vi "Config_Global.vi"() -> ()   [LabVIEW 2014]
panel:
  in  "Pod 3":T1
  in  "Pod 2":T1
  in  "Pod 1":T1
  in  "General":T2
  in  "Pod 0":T1
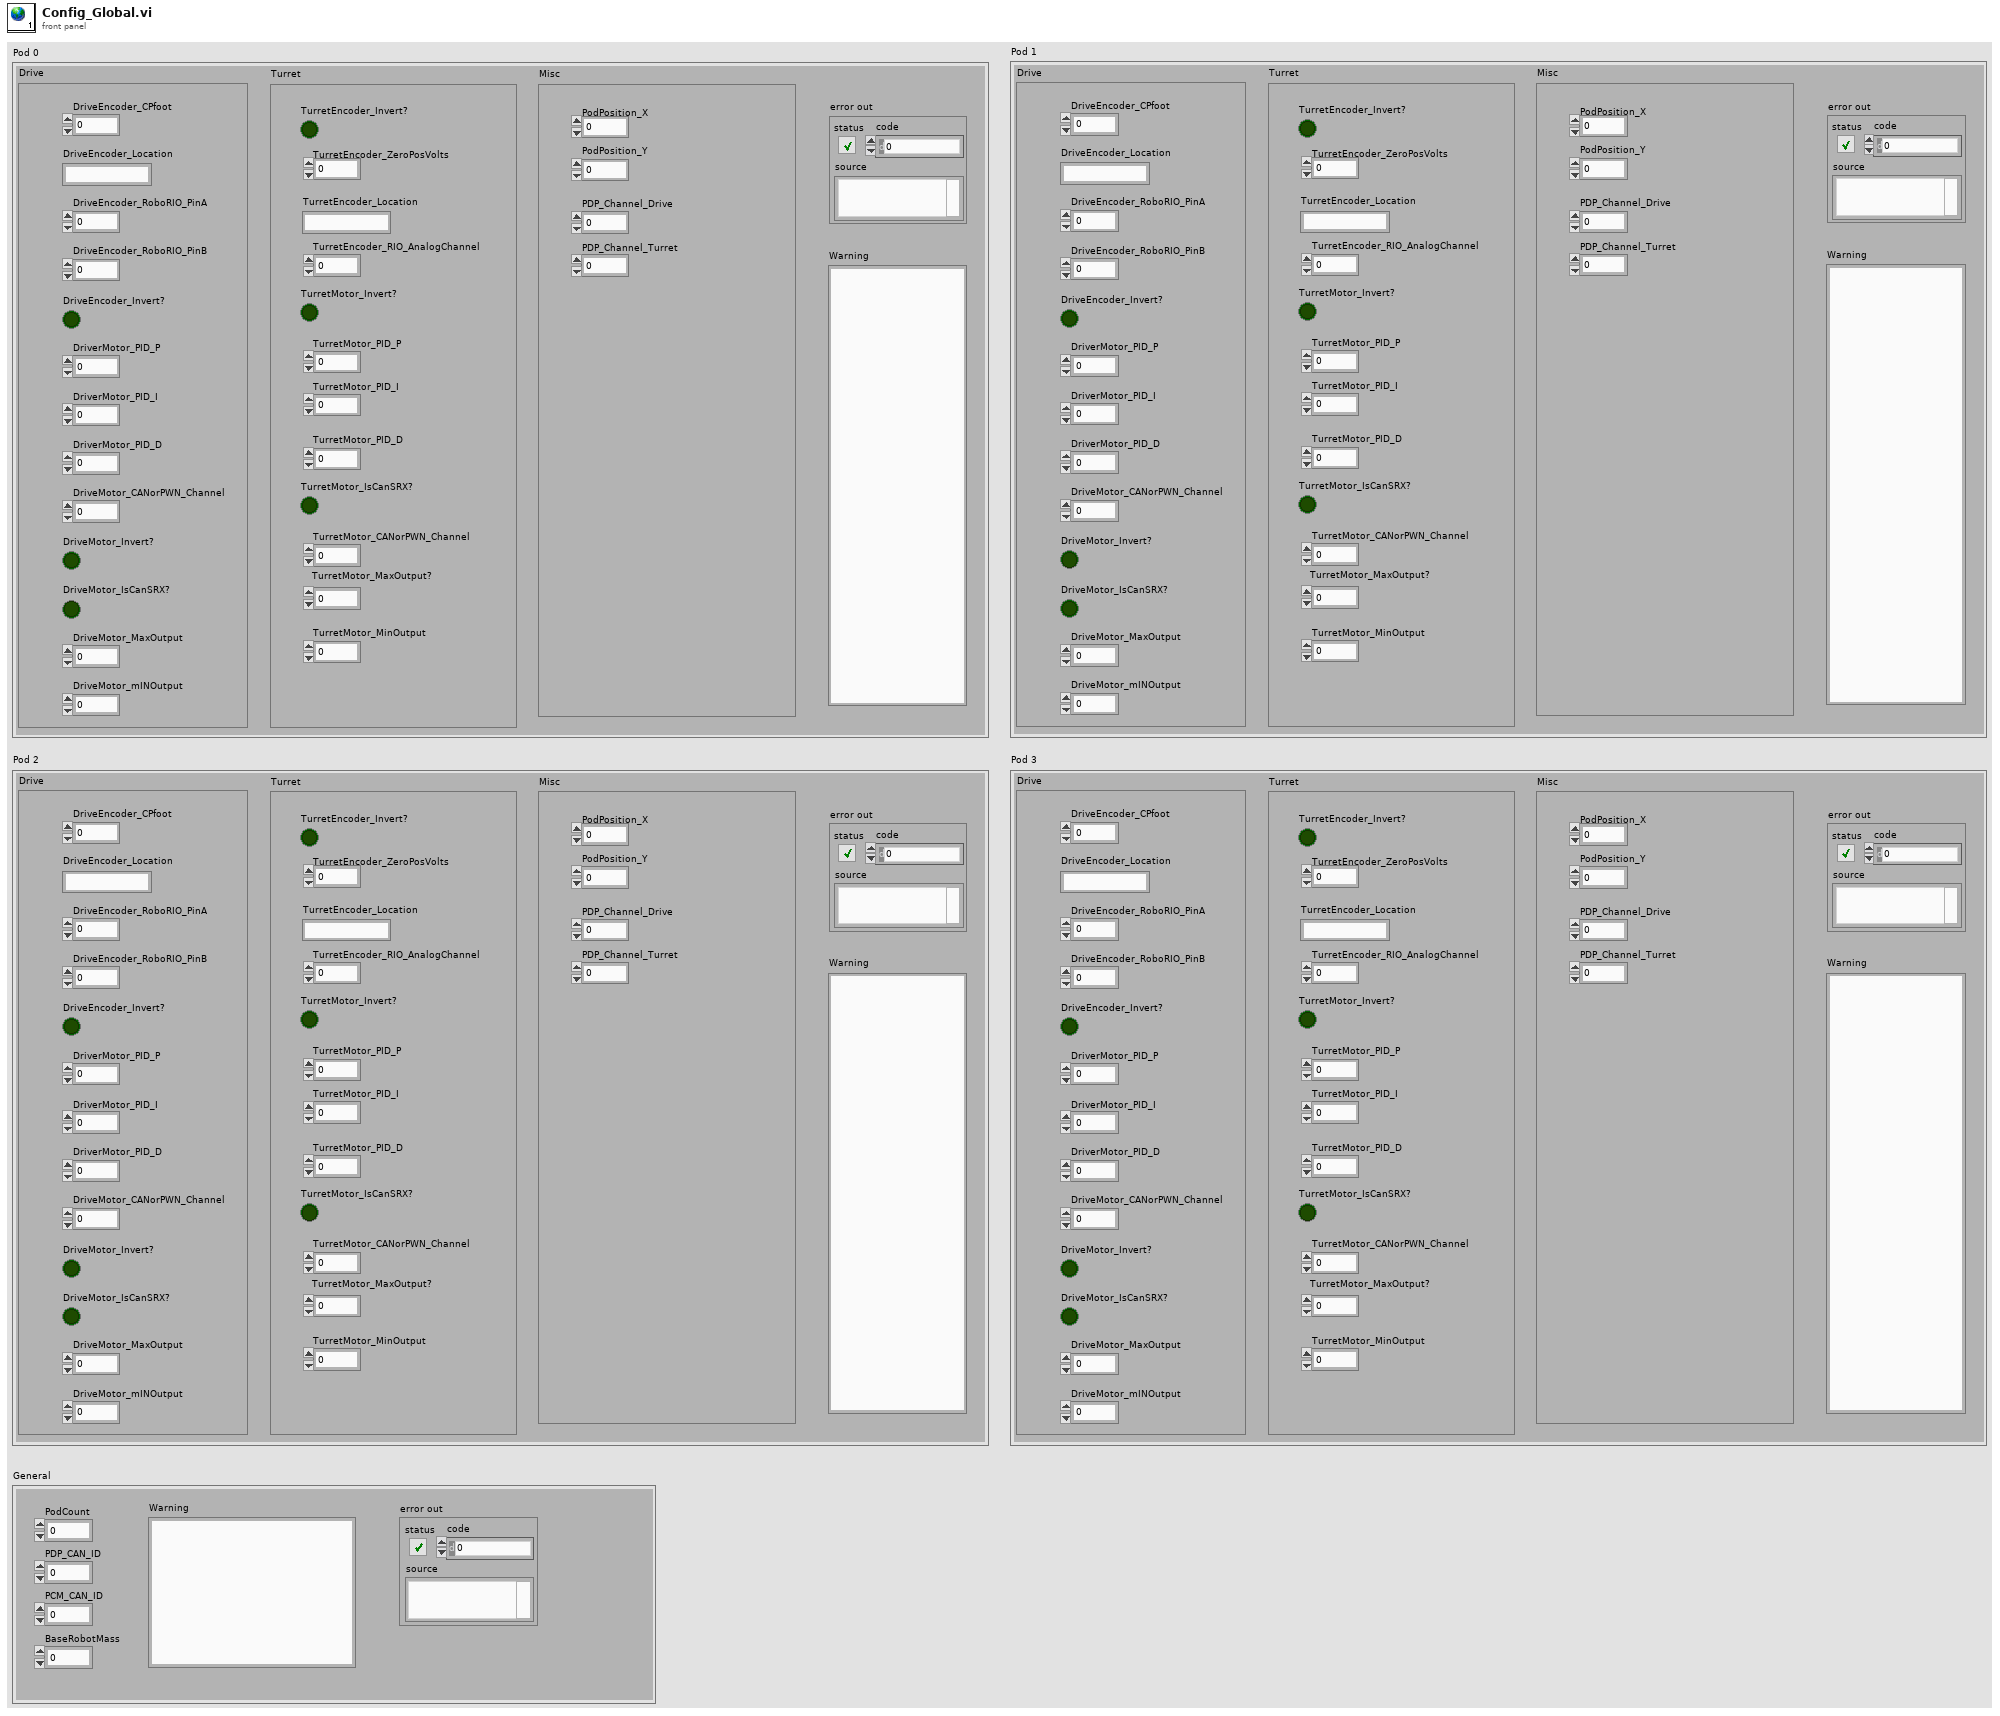
[diagram p1: front panel]
types:
  T1 = cluster{"Drive":cluster{"DriveEncoder_CPfoot":dbl, "DriveEncoder_Location":string, "DriveEncoder_RoboRIO_PinA":i32, "DriveEncoder_RoboRIO_PinB":i32, "DriveEncoder_Invert?":bool, "DriverMotor_PID_P":dbl, "DriverMotor_PID_I":dbl, "DriverMotor_PID_D":dbl, "DriveMotor_CANorPWN_Channel":i32, "DriveMotor_Invert?":bool, "DriveMotor_IsCanSRX?":bool, "DriveMotor_MaxOutput":dbl, "DriveMotor_mINOutput":dbl}, "Turret":cluster{"TurretEncoder_Invert?":bool, "TurretEncoder_ZeroPosVolts":dbl, "TurretEncoder_Location":string, "TurretEncoder_RIO_AnalogChannel":dbl, "TurretMotor_Invert?":bool, "TurretMotor_PID_P":dbl, "TurretMotor_PID_I":dbl, "TurretMotor_PID_D":dbl, "TurretMotor_CANorPWN_Channel":dbl, "TurretMotor_IsCanSRX?":bool, "TurretMotor_MaxOutput?":dbl, "TurretMotor_MinOutput":dbl}, "Misc":cluster{"PodPosition_X":dbl, "PodPosition_Y":dbl, "PDP_Channel_Drive":i32, "PDP_Channel_Turret":i32}, "error out":errorcluster, "Warning":string}
  T2 = cluster{"PodCount":dbl, "PDP_CAN_ID":i32, "PCM_CAN_ID":i32, "BaseRobotMass":dbl, "Warning":string, "error out":errorcluster}
diagram:
